vi "Check if pin is configured (SubVI).vi"(8 "error in (no error)":errorcluster, 10 "Pin in":u8, 11 "Lines":T1[](array[typedef]) items=["DIO1...8"=1, "DIO9...16"=2, "DIO17...24"=3, "DIO25...32"=4]) -> (0 "error out":errorcluster)   [LabVIEW 2009, in "MicroDAQ.lvlib" / "Digital Input.lvclass"]
uses:
  <instrlib>/MicroDAQ/Channel/Digital Input/Digital Input.lvclass
  <instrlib>/MicroDAQ/Tools/Digital IO channels.ctl
  <instrlib>/MicroDAQ/MicroDAQ.lvlib
panel:
  out "Pin is configured":bool
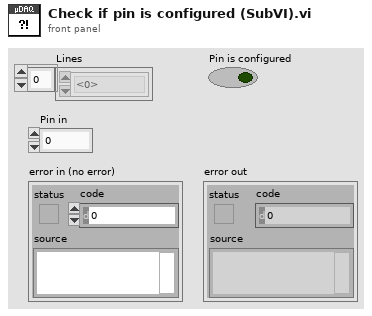
[diagram p1: front panel]
types:
  T1 = typedef "MicroDAQ.lvlib/Digital IO channels.ctl" = u8
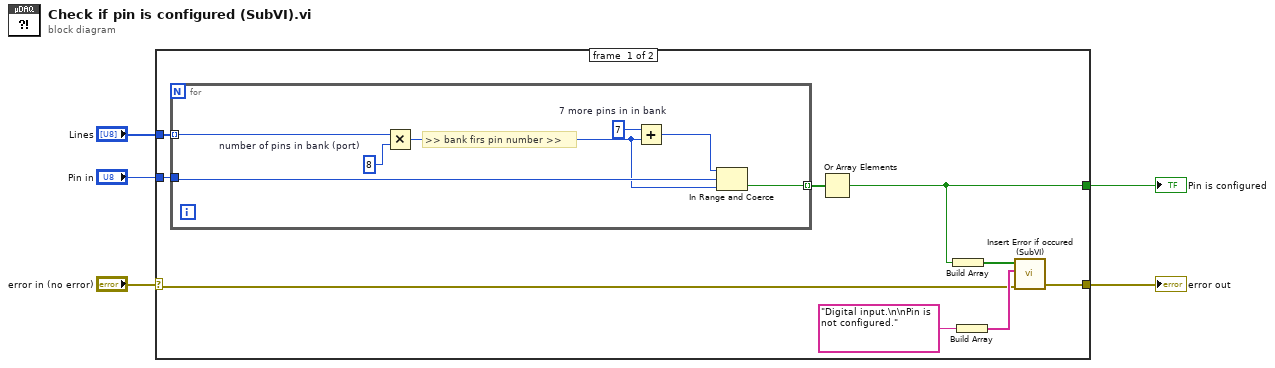
[diagram p0: block diagram]
diagram:
  n1 = case shown="No Error" "error in (no error)" {
    selector: "error in (no error)" -> [w9 w22]
    tunnel: [w6 _] -> w5
    tunnel: "Pin in" -> [w13 _]
    tunnel: "Lines" -> [w12 _]
    tunnel: [w8 w22] -> w1
    frame #0 {
      n2 = for {
        tunnel: w12 -> [w20] mode=indexing
        tunnel: w13 -> [w21]
        tunnel: [w15] -> w14 mode=indexing
        w18 = 7  # 7 more pins in in bank
        w19 = 8  # number of pins in bank (port)
        # ">> bank firs pin number >>"
        n3 = Multiply(x=w20, y=w19) -> (x*y=w16:i32)
        n4 = Add(x=w18, y=w16) -> (x+y=w17:i32)
        n5 = In Range and Coerce(upper limit=w17, x=w21, lower limit=w16) -> (In Range?=w15:bool)  [unwired: 1 out]
      }
      n6 = Or Array Elements(Boolean array=w14) -> (logical OR=w6:bool)
      n7 = Build Array(w6) -> (w7:bool[])
      n8 = Build Array("Digital input.\n\nPin is not configured.") -> (w11:string[])
      n9 = call <instrlib>:"Insert Error if occured (SubVI).vi"("error in (no error)"=w9, "Error messages"=w11, "Error conditionals"=w7) -> ("error out"=w8:errorcluster)  [unwired: 8 in]
    }
    frame #1 {
    }
  }
  "Pin is configured" <- w5
  "error out" <- w1
